vi "Test DVR Flatten.vi"() -> ()   [LabVIEW 2021]
uses:
  typedef/Datatype Waveform.ctl
  CIFChannels/CIFChannels.lvclass/CIFChannels.ctl
  <vilib>/CIF Foundation/CIF Utilities/DataTypes/Flatten U64.vi
  CIFChannels/Utilities/Create Flattened FIFO Header.vi
  Utilities/Unflatten Header.vi
  Utilities/Add Error.vi
  <vilib>/CIF Foundation/CIF Utilities/DataTypes/Unflatten U64.vi
  Utilities/Flatten Header.vi
  CIFChannels/Utilities/Update FIFO Header.vi
  <vilib>/CIF Foundation/CIF Utilities/DataTypes/Unflatten I64.vi
  <vilib>/CIF Foundation/CIF Utilities/Errors/Append Error Location.vi
  <vilib>/CIF Foundation/CIF Utilities/DataTypes/Flatten I64.vi
  <vilib>/CIF Foundation/CIF Utilities/Time/System Time/Get System Time.vi
  <vilib>/CIF Foundation/CIF Utilities/Time/System Time/LabVIEW Time to TAI Time.vi
  CIFChannels/CIFChannels.lvclass
  ChannelCommon.lvlib
panel:
  out "Array":T1[](array[typedef])
  out "Data out":u64[](array[numeric])
  out "error out":errorcluster
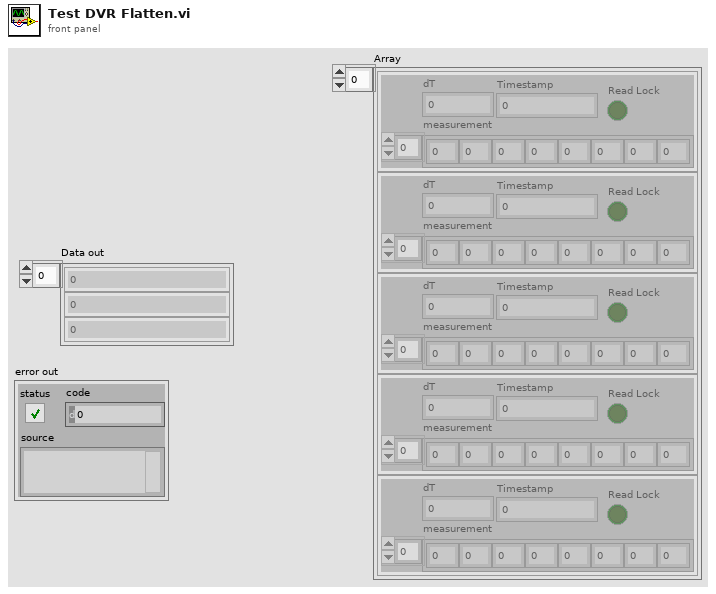
[diagram p1: front panel]
types:
  T1 = typedef "ChannelCommon.lvlib/Datatype Waveform.ctl" = cluster{"measurement":dbl[], "dT":dbl, "Timestamp":i64, "Read Lock":bool}
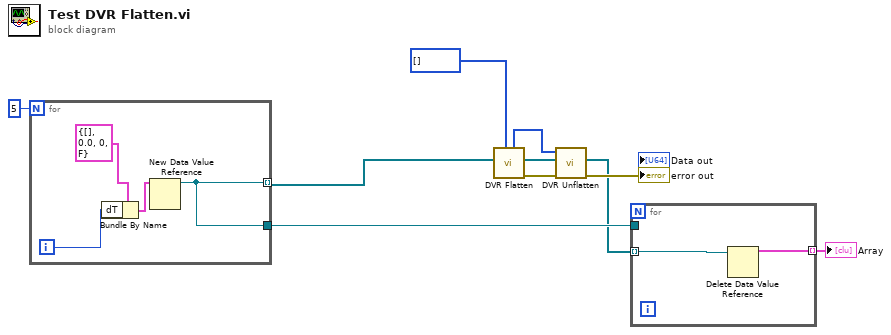
[diagram p0: block diagram]
diagram:
  n1 = for {
    N: 5 -> [_]
    tunnel: [w14] -> w2 mode=indexing
    tunnel: [w14] -> w4
    i -> [w12]
    n2 = Bundle By Name(cluster=T1 {"measurement"=[], "dT"=0.0, "Timestamp"=0, "Read Lock"=FALSE} ("Waveform Datatype"), "dT"=w12) -> (w11:T1)
    n3 = New Data Value Reference(data value=w11) -> (data value reference=w14:refnum<data-value>)  [unwired: 1 in, 1 out]
  }
  n4 = call "DVR Flatten.vi"("payload in"=u8[] [], "Data In"=w2) -> ("error out"=w10:errorcluster, "Data Out"=w6:refnum<data-value>[], "payload out"=w9:u8[])  [unwired: 5 in, 2 out]
  n5 = call "DVR Unflatten.vi"("error in (no error)"=w10, "DVRs In"=w6, "Flatten Data in"=w9) -> ("error out"=→"error out":errorcluster, "DVRs Out"=w3:refnum<data-value>[])  [unwired: 5 in, 2 out]
  n6 = for {
    tunnel: w3 -> [w15] mode=indexing
    tunnel: w4 -> [_]
    tunnel: [w16] -> w1 mode=indexing
    n7 = Delete Data Value Reference(data value reference=w15) -> (data value=w16:T1)  [unwired: 1 in, 1 out]
  }
  "Array" <- w1
